vi "Compressor No Cylinder shared.vi"() -> ()   [LabVIEW 2014]
doc: "Compressor with Cylinder \n\nThis example shows how to control a compressor, extend and retract a cylinder, and optionally use a limit switch to retract automatically.\n\nThis example works with the PCM (Pneumatic Control Module) communicating with the roboRIO over CAN bus. The PCM must also be supplied with 12V DC from the PDP (Power Distribution Panel).\n\nThe Compressor, Pressure Switch, and Solenoids are all wired to the PCM \n\nThe Limit Switch is wired to DIO 9. It causes the cylinder to retract when the Auto Retract button is pressed.\n\nRefer to the Pneumatics Manual for air connections. Your pneumatics setup should include a compressor, pressure switch, tank, regulator, valve, flow controls, cylinder, plug valve, etc.\n\nTo run this example you should have a pneumatic system with air pressure connected to the P input on the SMC double solenoid valve. The A output of the valve should be connected via a flow control to the backend of a cylinder. The B output of the valve should be connected via a flow control to the frontend of a cylinder. When the cylinder is extended, it should physically depress the Limit Switch.\n\nWith the VI running, pressing the Extend button will push the cylinder shaft out, and pressing the Retract button will pull it back. Notice that the Extend and Retract buttons have their Mechanical Action set to Latch When Pressed. This means they stay pressed (ON) until they are read by the program, then they return to the OFF position. This works because once the SMC solenoid valve is pulled one direction, it stays in that position until it is pulled in the opposite direction - it only needs to be momentarily energized. The Auto Retract button can be used to make the cylinder return automatically. With the Auto Retract button ON, pressing the Extend button will push the cylinder out, and it will retract when it hits the limit switch.\n\nThis example expects a USB cable connected from your development PC to the Type B USB Jack (next to the power input) on the roboRIO.\n\nThis example expects the Driver Station to be running."
panel:
  out "Compressor Running":bool
  out "Compressor Monitoring":bool
  in  "stop":bool
  # "Set these inputs before running."
  # "roboRIO Wiring Diagram"
  # "when extended, the cylinder should depress this"
  # "Limit\nSwitch"
  # "These can be set while running."
  # "Pneumatic Control Module Wiring Diagram"
  # "Output information."
  # "Connect\nPower in\nHere"
  # "Connect\nCompressor\nHere"
  # "tubing port for retract side of cylinder"
  # "tubing port for extend side of cylinder"
  # "Pressure\nSwitch"
  # "SMC double solenoid valve"
  # "CAN"
  # "COMPRESSOR OUT"
  # "PRESSURE"
  # "NC"
  # "C"
  # "B"
  # "A"
  # "B"
  # "A"
  # "COM"
  # "NC"
  # "NO"
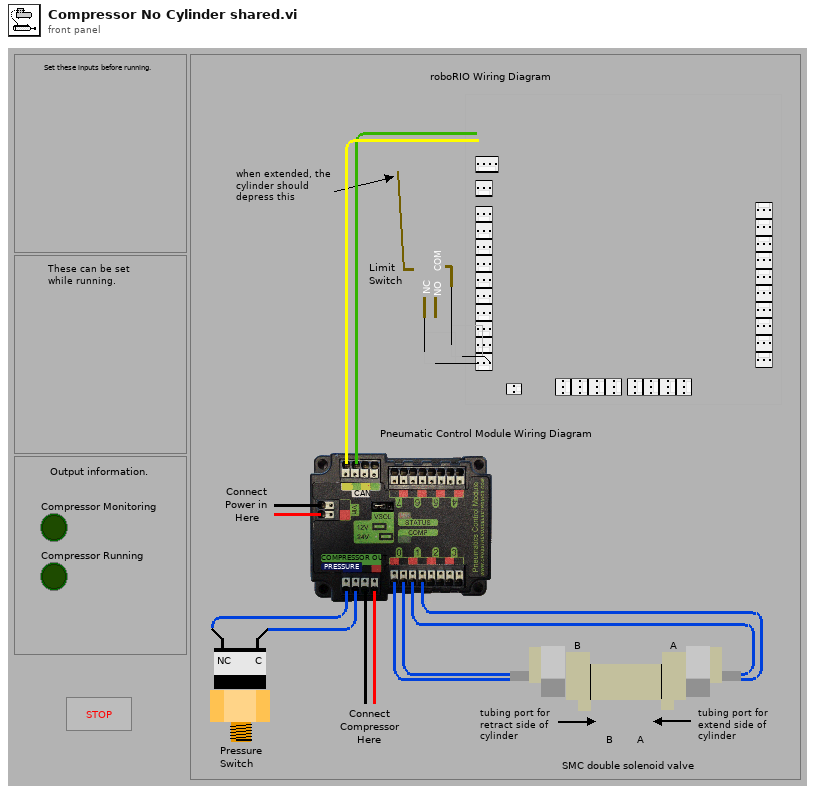
[diagram p1: front panel]
types:
  T1 = typedef "WPI_CompressorDevRef.ctl" = cluster{"DevStatus":errorcluster, "Pneumatics Control Module":u8}
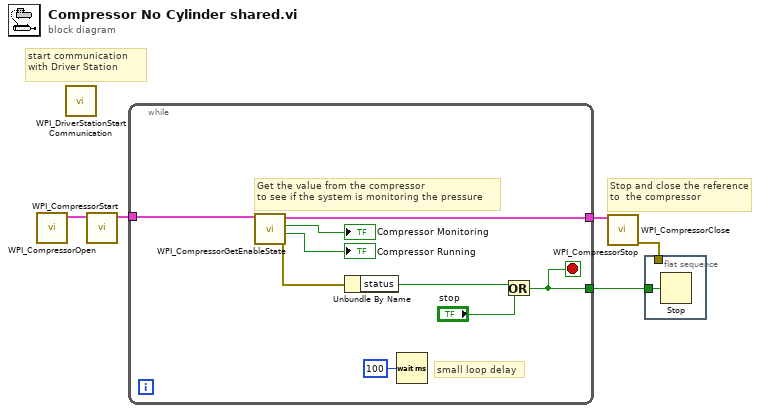
[diagram p0: block diagram]
diagram:
  # "start communication with Driver Station"
  # "Stop and close the reference to  the compressor"
  n1 = call <vilib>:"WPI_CompressorOpen.vi"() -> ("CompressorDevRef"=w3:T1)  [unwired: 14 in, 1 out]
  n2 = call <vilib>:"WPI_DriverStationStart Communication.vi"() -> ()  [unwired: 2 in, 10 out]
  n3 = call <vilib>:"WPI_CompressorStart.vi"("CompressorDevRef"=w3) -> ("CompressorDevRef"=w5:T1)  [unwired: 1 in, 9 out]
  n4 = while {
    tunnel: w5 -> [w15]
    tunnel: [w14] -> w4
    tunnel: [w12] -> w2
    stop <- w12 stop-if-true
    # "small loop delay"
    # "Get the value from the compressor \nto see if the system is monitoring the pressure"
    n5 = call <vilib>:"WPI_CompressorGetEnableState.vi"("CompressorDevRef"=w15) -> ("error out"=w10:errorcluster, "Compressor Running"=→"Compressor Running":bool, "Enabled"=→"Compressor Monitoring":bool, "CompressorDevRef"=w14:T1)  [unwired: 1 in, 6 out]
    n6 = Unbundle By Name(w10) -> ("status"=w9:bool)
    n7 = Wait (ms)(milliseconds to wait=u32 100) -> ()  [unwired: 1 out]
    n8 = Or(x=w9, y="stop") -> (x .or. y?=w12:bool)
  }
  n9 = call <vilib>:"WPI_CompressorStop.vi"("CompressorDevRef"=w4) -> ("CompressorDevRef"=w6:T1)  [unwired: 1 in, 9 out]
  n10 = call <vilib>:"WPI_CompressorClose.vi"("CompressorDevRef"=w6) -> ("error out"=w1:errorcluster)  [unwired: 1 in, 9 out]
  n11 = flat-sequence {
    tunnel: w2 -> [w16]
    tunnel: w1 -> [_]
    frame #0 {
      n12 = Stop(stop? (T)=w16) -> ()
    }
  }
